vi "Send Packet.vi"(6 "timeout (0ms : no ack)":i32, 8 "error in (no error)":errorcluster, 10 "Packet":refnum<class "ControlPacket.lvclass">, 11 "Session":refnum<class "Session.Client.lvclass">) -> (0 "error out":errorcluster, 1 "validated":bool, 2 "Response":refnum<class "ControlPacket.lvclass">[](array[class]), 3 "Session":refnum<class "Session.Client.lvclass">)   [LabVIEW 2013, in "MQTT Client.lvlib" / "Session.Client.lvclass"]
uses:
  Session.Client.lvclass
  <vilib>/LabVIEW Open Source Project/MQTT Control Packets/Control Packets/ControlPacket/ControlPacket.lvclass
  <vilib>/LabVIEW Open Source Project/MQTT Connection/MQTT_Base/Base Class/Response -- cluster.ctl
  <vilib>/LabVIEW Open Source Project/MQTT Connection/MQTT_Base/Session/Session.lvclass/Session.ctl
  <vilib>/LabVIEW Open Source Project/MQTT Connection/MQTT_Base/Base Class/MQTT_Base.lvclass
  <vilib>/LabVIEW Open Source Project/MQTT Connection/MQTT_Base/Session/Session.lvclass
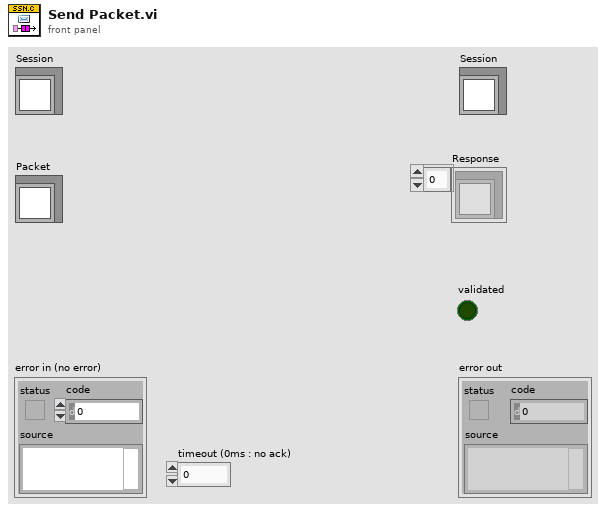
[diagram p1: front panel]
types:
  T1 = typedef "MQTT Base.lvlib/MQTT_Base.lvclass/Response -- cluster.ctl" = cluster{"Packet":refnum<class "ControlPacket.lvclass">, "Protocol Error":errorcluster, "disconnect session":bool, "[ACK]":refnum<notifier>[]}
  T2 = typedef "MQTT_Control_Packets.lvlib/ControlPacket.lvclass/Control Packet Type -- enum.ctl" = enum16{"Reserved", "CONNECT", "CONNACK", "PUBLISH", "PUBACK", "PUBREC", "PUBREL", "PUBCOMP", "SUBSCRIBE", "SUBACK", "UNSUBSCRIBE", "UNSUBACK", "PINGREQ", "PINGRESP", "DISCONNECT", "AUTH"}
  T3 = typedef "MQTT_Control_Packets.lvlib/ControlPacket.lvclass/QualityOfService -- enum.ctl" = enum16{"0 (At Most Once)", "1 (At Least Once)", "2 (Exactly Once)"}
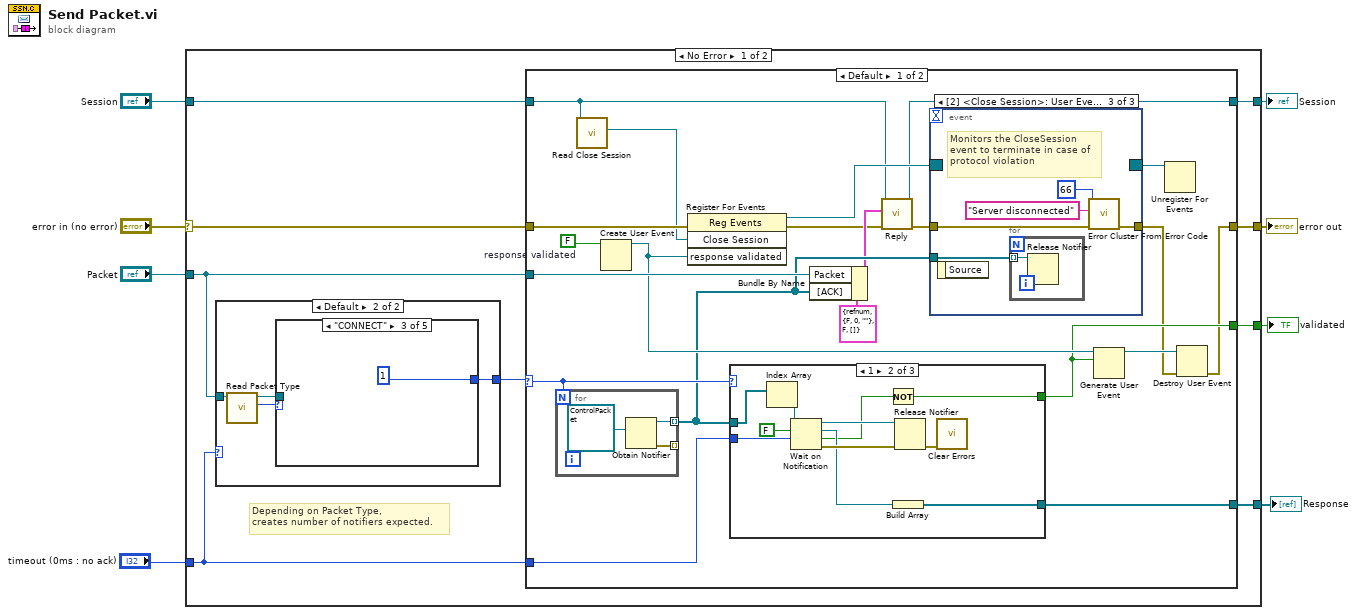
[diagram p0: block diagram]
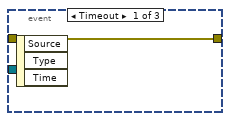
[diagram p2: hidden frame]
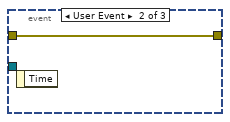
[diagram p3: hidden frame]
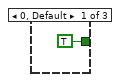
[diagram p4: hidden frame]
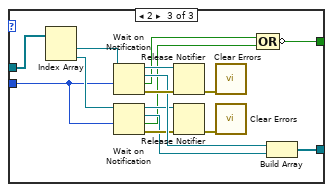
[diagram p5: hidden frame]
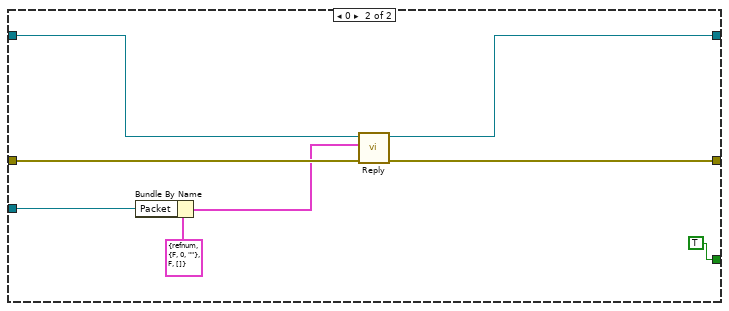
[diagram p6: hidden frame]
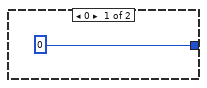
[diagram p7: hidden frame]
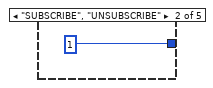
[diagram p9: hidden frame]
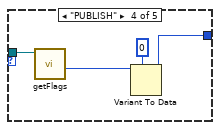
[diagram p10: hidden frame]
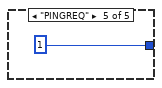
[diagram p11: hidden frame]
diagram:
  n1 = case shown="No Error" "error in (no error)" {
    selector: "error in (no error)" -> [w12 w99]
    tunnel: [w11 w99] -> w7
    tunnel: [w10 w98] -> w5
    tunnel: "Session" -> [w16 w98]
    tunnel: "Packet" -> [w17 _]
    tunnel: [w13 _] -> w3
    tunnel: "timeout (0ms : no ack)" -> [w15 _]
    tunnel: [w14 _] -> w1
    frame No Error {
      # "Depending on Packet Type, \ncreates number of notifiers expected."
      n2 = case shown="Default" w15 {
        tunnel: w17 -> [_ w90]
        tunnel: [0 w87] -> w9
        frame 0 {
        }
        frame Default {
          n3 = call <vilib>:"Read Packet Type.vi"("ControlPacket in"=w90) -> ("Control Packet Type"=w88:T2, "ControlPacket out"=w89:refnum<class "ControlPacket.lvclass">)  [unwired: 9 in]
          n4 = case shown="\"CONNECT\"" w88 {
            tunnel: w89 -> [_ _ _ w95 _]
            tunnel: [_ 1 1 w94 1] -> w87
            frame Default {
            }
            frame "SUBSCRIBE", "UNSUBSCRIBE" {
            }
            frame "CONNECT" {
            }
            frame "PUBLISH" {
              n5 = call-dynamic "getFlags.vi"("ControlPacket in"=w95) -> ("QoS"=w93:T3)  [unwired: 7 in, 3 out]
              n6 = Variant To Data(type=0, Variant=w93) -> (data=w94:i32)  [unwired: 1 in, 1 out]
            }
            frame "PINGREQ" {
            }
          }
        }
      }
      n7 = case shown="Default" w9 {
        selector: w9 -> [w34 _]
        tunnel: w17 -> [w38 w85]
        tunnel: w16 -> [w19 w79]
        tunnel: w15 -> [w36 _]
        tunnel: [w35 _] -> w14
        tunnel: [w30 TRUE] -> w13
        tunnel: w12 -> [w33 w82]
        tunnel: [w26 w81] -> w11
        tunnel: [w23 w78] -> w10
        frame Default {
          w32 = FALSE  # response validated
          n8 = for {
            N: w34 -> [_]
            tunnel: [w77] -> _ mode=indexing
            tunnel: [w76] -> w24 mode=indexing
            n9 = Obtain Notifier(notification data type=refnum<class "ControlPacket.lvclass"> refnum ("Ack")) -> (notifier out=w76:refnum<notifier>, error out=w77:errorcluster)  [unwired: 3 in, 1 out]
          }
          n10 = call <vilib>:"Read Close Session.vi"("Session in"=w19) -> ("Close Session"=w18:refnum<user-event>)  [unwired: 8 in, 2 out]
          n11 = Create User Event(user event datatype=w32) -> (user event=w31:refnum<user-event>)  [unwired: 1 in, 1 out]
          n12 = register-events(error in=w33, w18, w31) -> (reference out=w29:refnum<event-registration>, error out=w21:errorcluster)  [unwired: 1 in]
          n13 = case shown="1" w34 {
            tunnel: w36 -> [_ w58 w62]
            tunnel: w24 -> [_ w53 w71]
            tunnel: [_ w50 w68] -> w35
            tunnel: [TRUE w48 w59] -> w30
            frame 0, Default {
            }
            frame 1 {
              n14 = Index Array(array=w53) -> (element=w52:refnum<notifier>)  [unwired: 1 in]
              n15 = Wait on Notification(notifier=w52, ignore previous (F)=FALSE, timeout in ms (-1)=w58) -> (notifier out=w55:refnum<notifier>, notification=w54:refnum<class "ControlPacket.lvclass">, timed out?=w49:bool, error out=w56:errorcluster)  [unwired: 1 in]
              n16 = Not(x=w49) -> (.not. x?=w48:bool)
              n17 = Build Array(w54) -> (w50:refnum<class "ControlPacket.lvclass">[])
              n18 = Release Notifier(notifier=w55, error in (no error)=w56) -> (error out=w51:errorcluster)  [unwired: 1 in, 2 out]
              n19 = call <vilib>:"Clear Errors.vi"("error in (no error)"=w51) -> ()  [unwired: 6 in, 1 out]
            }
            frame 2 {
              n20 = Index Array(array=w71) -> (element #1=w70:refnum<notifier>, element #2=w64:refnum<notifier>)  [unwired: 2 in]
              n21 = Wait on Notification(notifier=w70, timeout in ms (-1)=w62) -> (notifier out=w73:refnum<notifier>, notification=w72:refnum<class "ControlPacket.lvclass">, timed out?=w61:bool, error out=w74:errorcluster)  [unwired: 2 in]
              n22 = Wait on Notification(notifier=w64, timeout in ms (-1)=w62) -> (notifier out=w63:refnum<notifier>, notification=w65:refnum<class "ControlPacket.lvclass">, timed out?=w60:bool, error out=w66:errorcluster)  [unwired: 2 in]
              n23 = Release Notifier(notifier=w73, error in (no error)=w74) -> (error out=w69:errorcluster)  [unwired: 1 in, 2 out]
              n24 = Release Notifier(notifier=w63, error in (no error)=w66) -> (error out=w67:errorcluster)  [unwired: 1 in, 2 out]
              n25 = call <vilib>:"Clear Errors.vi"("error in (no error)"=w69) -> ()  [unwired: 6 in, 1 out]
              n26 = call <vilib>:"Clear Errors.vi"("error in (no error)"=w67) -> ()  [unwired: 6 in, 1 out]
              n27 = Compound Arithmetic op=OR(w61, w60) -> (invert w59:bool)
              n28 = Build Array(w72, w65) -> (w68:refnum<class "ControlPacket.lvclass">[])
            }
          }
          n29 = Bundle By Name(cluster=T1 {"Packet"=refnum, "Protocol Error"={"status"=FALSE, "code"=0, "source"=""}, "disconnect session"=FALSE, "[ACK]"=[]} ("element"), "Packet"=w38, "[ACK]"=w24) -> (w22:T1)
          n30 = call <vilib>:"Reply.vi"("error in (no error)"=w21, "Outgoing Element"=w22, "Session in"=w19) -> ("error out"=w20:errorcluster, "Session out"=w23:refnum<class "Session.Client.lvclass">)  [unwired: 7 in]
          n31 = event shown="[2] <Close Session>: User Event" {
            selector: w29 -> [_ _ _]
            dyn-events: [_ _ _] -> w28
            timeout: _ -> [_ _ _]
            tunnel: w20 -> [w39 w40 w43]
            tunnel: [w39 w40 w44] -> w25
            tunnel: w24 -> [_ _ w45]
            event Timeout {
              n32 = event-data() -> ()  [unwired: 1 in, 3 out]
            }
            event User Event {
              n33 = event-data() -> ()  [unwired: 1 in, 1 out]
            }
            event User Event {
              # "Monitors the CloseSession\nevent to terminate in case of\nprotocol violation"
              n34 = event-data() -> ()  [unwired: 1 in, 1 out]
              n35 = for {
                tunnel: w45 -> [w46] mode=indexing
                n36 = Release Notifier(notifier=w46) -> ()  [unwired: 2 in, 3 out]
              }
              n37 = call <vilib>:"Error Cluster From Error Code.vi"("error in (no error)"=w43, "error message (\"\")"="Server disconnected" ("error message (\"\")"), "error code (0)"=66) -> ("error out"=w44:errorcluster)  [unwired: 6 in]
            }
          }
          n38 = Generate User Event(user event=w31, event data cluster=w30) -> (user event out=w27:refnum<user-event>)  [unwired: 2 in, 1 out]
          n39 = Unregister For Events(event registration refnum=w28) -> ()  [unwired: 1 in, 1 out]
          n40 = Destroy User Event(user event=w27, error in=w25) -> (error out=w26:errorcluster)
        }
        frame 0 {
          n41 = Bundle By Name(cluster=T1 {"Packet"=refnum, "Protocol Error"={"status"=FALSE, "code"=0, "source"=""}, "disconnect session"=FALSE, "[ACK]"=[]} ("element"), "Packet"=w85) -> (w80:T1)
          n42 = call <vilib>:"Reply.vi"("error in (no error)"=w82, "Outgoing Element"=w80, "Session in"=w79) -> ("error out"=w81:errorcluster, "Session out"=w78:refnum<class "Session.Client.lvclass">)  [unwired: 7 in]
        }
      }
    }
    frame Error {
    }
  }
  "error out" <- w7
  "Session" <- w5
  "validated" <- w3
  "Response" <- w1
